vi "Read STOPPED.vi"(8 "error in (no error)":errorcluster, 11 "Monkey in":refnum<class "Tamer.lvclass">) -> (0 "error out":errorcluster, 2 "STOPPED":bool, 3 "Monkey out":refnum<class "Tamer.lvclass">)   [LabVIEW 2020, in "Tamer.lvlib" / "Tamer.lvclass"]
uses:
  Tamer.lvclass
  Tamer.lvclass/Tamer.ctl
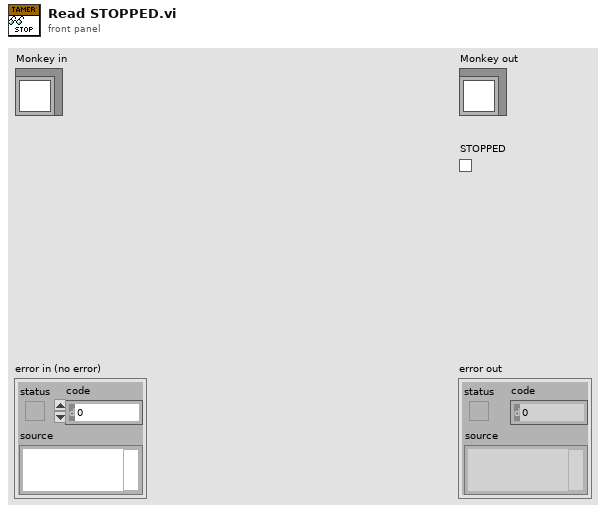
[diagram p1: front panel]
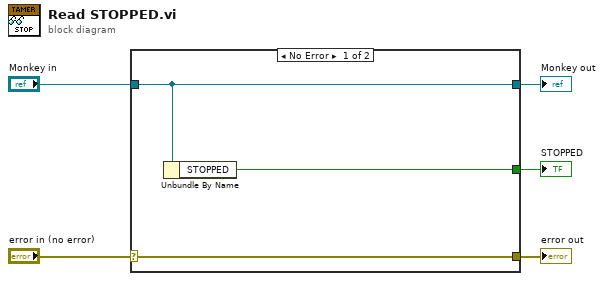
[diagram p0: block diagram]
diagram:
  n1 = case shown="No Error" "error in (no error)" {
    selector: "error in (no error)" -> [w8 w9]
    tunnel: [w8 w9] -> w4
    tunnel: [w7 w10] -> w2
    tunnel: "Monkey in" -> [w7 w10]
    tunnel: [w6 _] -> w1
    frame No Error {
      n2 = Unbundle By Name(w7) -> ("STOPPED"=w6:bool)
    }
    frame Error {
    }
  }
  "error out" <- w4
  "Monkey out" <- w2
  "STOPPED" <- w1
